vi "Find Implementation.vi"(3 "error in":errorcluster, 4 "Method Name":string, 5 "Class in":refnum<vi>) -> (0 "error out":errorcluster, 1 "VI":refnum<vi>, 2 "Class out":refnum<vi>)   [LabVIEW 2020, in "Choose Implementation Dialog.lvlib"]
uses:
  Choose Implementation Dialog.lvlib
  3ece226a-d8ec-49aa-a75f-05626d7b5125.vi
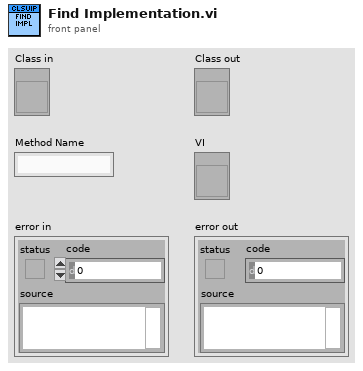
[diagram p1: front panel]
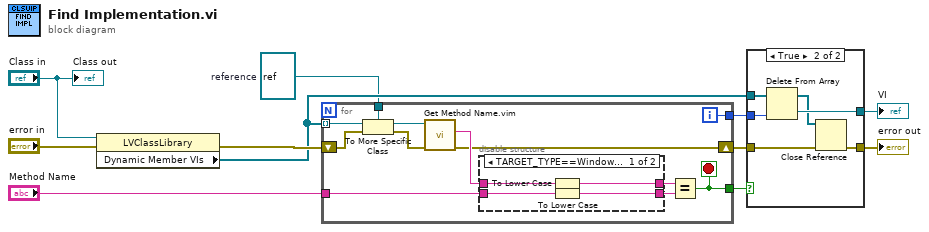
[diagram p0: block diagram]
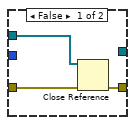
[diagram p2: hidden frame]
diagram:
  w1 = refnum<vi> refnum  # reference
  n1 = property class="LVClassLibrary"(reference="Class in", error in="error in") -> (error out=w9:errorcluster, "Dynamic Member VIs"=w4:refnum<vi>[])  [unwired: 1 out]
  n2 = for {
    shift-right: [w21] -> w5
    shift-left: w9 -> [w13]
    tunnel: w4 -> [w16] mode=indexing
    tunnel: "Method Name" -> [w22]
    tunnel: [w18] -> w6
    tunnel: [w17] -> w7
    tunnel: w1 -> [w14]
    i -> [w17]
    stop <- w18 stop-if-true
    n3 = To More Specific Class(target class=w14, reference=w16, error in=w13) -> (specific class reference=w15:refnum<vi>, error out=w12:errorcluster)
    n4 = call "Get Method Name.vim"("error in (no error)"=w12, "VI Reference/Name"=w15) -> ("error out"=w21:errorcluster, "Method Name"=w23:string)  [unwired: 7 in, 1 out]
    n5 = disable-structure shown="TARGET_TYPE==Windows" {
      disable-tunnel: w23 -> [w27 w29]
      disable-tunnel: w22 -> [w26 w28]
      disable-tunnel: [w25 w29] -> w20
      disable-tunnel: [w24 w28] -> w19
      frame condition #0 (active) {
        n6 = To Lower Case(string=w27) -> (all lower case string=w25:string)
        n7 = To Lower Case(string=w26) -> (all lower case string=w24:string)
      }
      frame condition #1 {
      }
    }
    n8 = Equal?(x=w20, y=w19) -> (x = y?=w18:bool)
  }
  n9 = case shown="True" w6 {
    tunnel: w7 -> [_ w36]
    tunnel: w5 -> [w32 w35]
    tunnel: w4 -> [w31 w38]
    tunnel: [w30 w34] -> w3
    tunnel: [_ w37] -> w2
    frame False {
      n10 = Close Reference(reference=w31, error in (no error)=w32) -> (error out=w30:errorcluster)
    }
    frame True {
      n11 = Delete From Array(array=w38, index=w36) -> (deleted portion=w37:refnum<vi>, array with subset deleted=w33:refnum<vi>[])  [unwired: 1 in]
      n12 = Close Reference(reference=w33, error in (no error)=w35) -> (error out=w34:errorcluster)
    }
  }
  "VI" <- w2
  "error out" <- w3
  "Class out" <- "Class in"
